vi "GV frameclock.vi"() -> ()   [LabVIEW 2017]
panel:
  out "Frameclock":bool
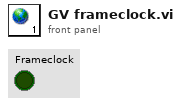
[diagram p1: front panel]
diagram:
